vi "DetectorVI.vi"(8 "error in":errorcluster, 9 "Visible Temp Controls":bool=TRUE, 10 "ControlQueue":refnum<queue>, 11 "Detector.lvclass":refnum<class "Detector.lvclass">) -> (0 "error out":errorcluster)   [LabVIEW 2015, in "Detector.lvclass"]
uses:
  Detector.lvclass
  controls/SliderSD.ctl
  dependecies/ControlsVIs/Clusters-def/Message types.ctl
  Controls-refs_CLIENT.ctl
  Detector.lvclass/Detector.ctl
  GeneralFunctionality/GeneralFunctionality.lvclass/GeneralFunctionality.ctl
  Message/Message.lvclass/Message.ctl
  dependecies/ControlsVIs/Clusters-def/Standard Command.ctl
  dependecies/ControlsVIs/Clusters-def/DAQmx-ELYSE_pulse_counter.ctl
  dependecies/ControlsVIs/Clusters-def/OSc-WCM_max_value.ctl
  dependecies/ControlsVIs/Clusters-def/OSc-Diodes.ctl
  dependecies/ControlsVIs/Clusters-def/Det-Read.ctl
  dependecies/ControlsVIs/Clusters-def/Parameters_measurement_def.ctl
  Write SC sum values ref.vi
  dependecies/globalVarII.vi
  Message/Message.lvclass
  Control/Control-Client/Control-Client.lvclass
  GeneralFunctionality/GeneralFunctionality.lvclass
  DAQmxTasks/DAQmxTaskContainer_General/DAQmxTaksContainer_General.lvclass
  Oscilloscope/Oscilloscope.lvclass
panel:
  in  "Tab Control":enum32{"Detector", "PhotoDiodes"}(tab)
  in  "waves slider":T1={434.19354838709677, 734.8387096774194} scale=240.824..813.9446 scale format="%#.1f"
  in  "# error":i32=10
  out "Error Meter":dbl(knob) scale=0.0..10.0
  out "#PP":i32
  out "Spectra":cluster{"wavelengths":dbl[], "Tableau":dbl[]}[](graph)
  out "OD":cluster{"wavelengths":dbl[], "Tableau":dbl[]}(graph)
  in  "BG-level":i32
  in  "SC sum values":i32[](array[numeric])
  in  "Zeros for VIS-NIR":i32
  in  "Save spectra":bool
  out "Termometer":i32(slide) caption="T, °C" scale=-50.0..50.0
  in  "Set T":i32=-35
  in  "ON/OFF Cool":bool
  out "delta O.D.":dbl
  out "Ref I0":dbl(slide) scale=0.0..10.0
  out "Signal I0":dbl(slide) scale=0.0..10.0
  out "Ref Ie":dbl(slide) scale=0.0..10.0
  out "Signal Ie":dbl(slide) scale=0.0..10.0
  in  "All":bool
  out "class name":string
  out "WCM max":dbl
  out "ELYSE pulses":dbl
  in  "# scans":i32=5 min=1 max=50 step=1
  in  "Read detector":bool
  out "Received command":string
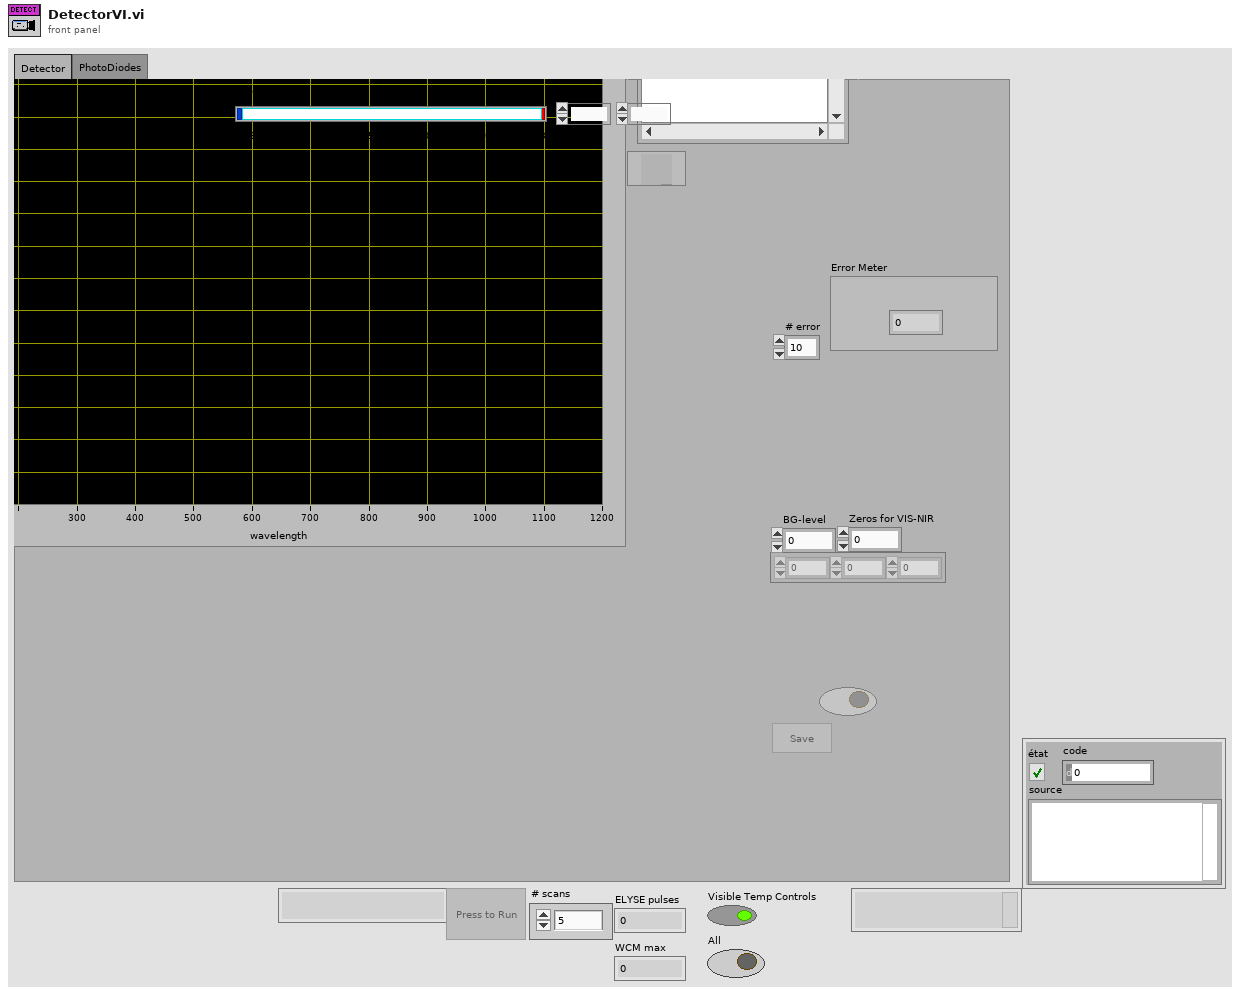
[diagram p1: front panel]
types:
  T1 = typedef "SliderSD.ctl" = cluster{dbl, dbl}
  T2 = typedef "Message types.ctl" = string
  T3 = typedef "Control-Client.lvclass/Controls-refs_CLIENT.ctl" = cluster{"ON/OFF Cool":refnum<vi>, "Save spectra":refnum<vi>, "Read detector":refnum<vi>, "# scans":refnum<vi>, "BG-level":refnum<vi>, "Set T":refnum<vi>, "Termometer":refnum<vi>, "Spectra":refnum<vi>, "Error Meter_ref":refnum<vi>, "waves slider":refnum<vi>}
  T4 = typedef "Standard Command.ctl" = cluster{"command":string, "data":variant}
  T5 = typedef "DAQmxTaksContainer_General.lvclass/DAQmx-ELYSE_pulse_counter.ctl" = cluster{"# counts":dbl}
  T6 = typedef "Oscilloscope.lvclass/OSc-WCM_max_value.ctl" = cluster{"WCM_max_value":dbl}
  T7 = typedef "Oscilloscope.lvclass/OSc-Diodes.ctl" = cluster{"I0":dbl, "Ie":dbl, "II0":dbl, "IIe":dbl, "BGI0":dbl, "BGIe":dbl, "BGII0":dbl, "BGIIe":dbl}
  T8 = typedef "Detector.lvclass/Det-Read.ctl" = cluster{"# scans":i32, "All":bool, "Parameters of measurement":T9}
  T9 = typedef "Parameters_measurement_def.ctl" = cluster{"ODmin":dbl, "ODmax":dbl, "Aq contol":enum32{"fixed", "automatic", "fixed-auto"}, "Wavelength_fix_index":i32, "WCM_limits":cluster{"WCM_min":dbl, "WCM_max":dbl, "WCM_value":dbl}, "WCM_corrections":bool, "#cycles max":i32}
  T10 = cluster{"closest index":i32, "closest index":i32}
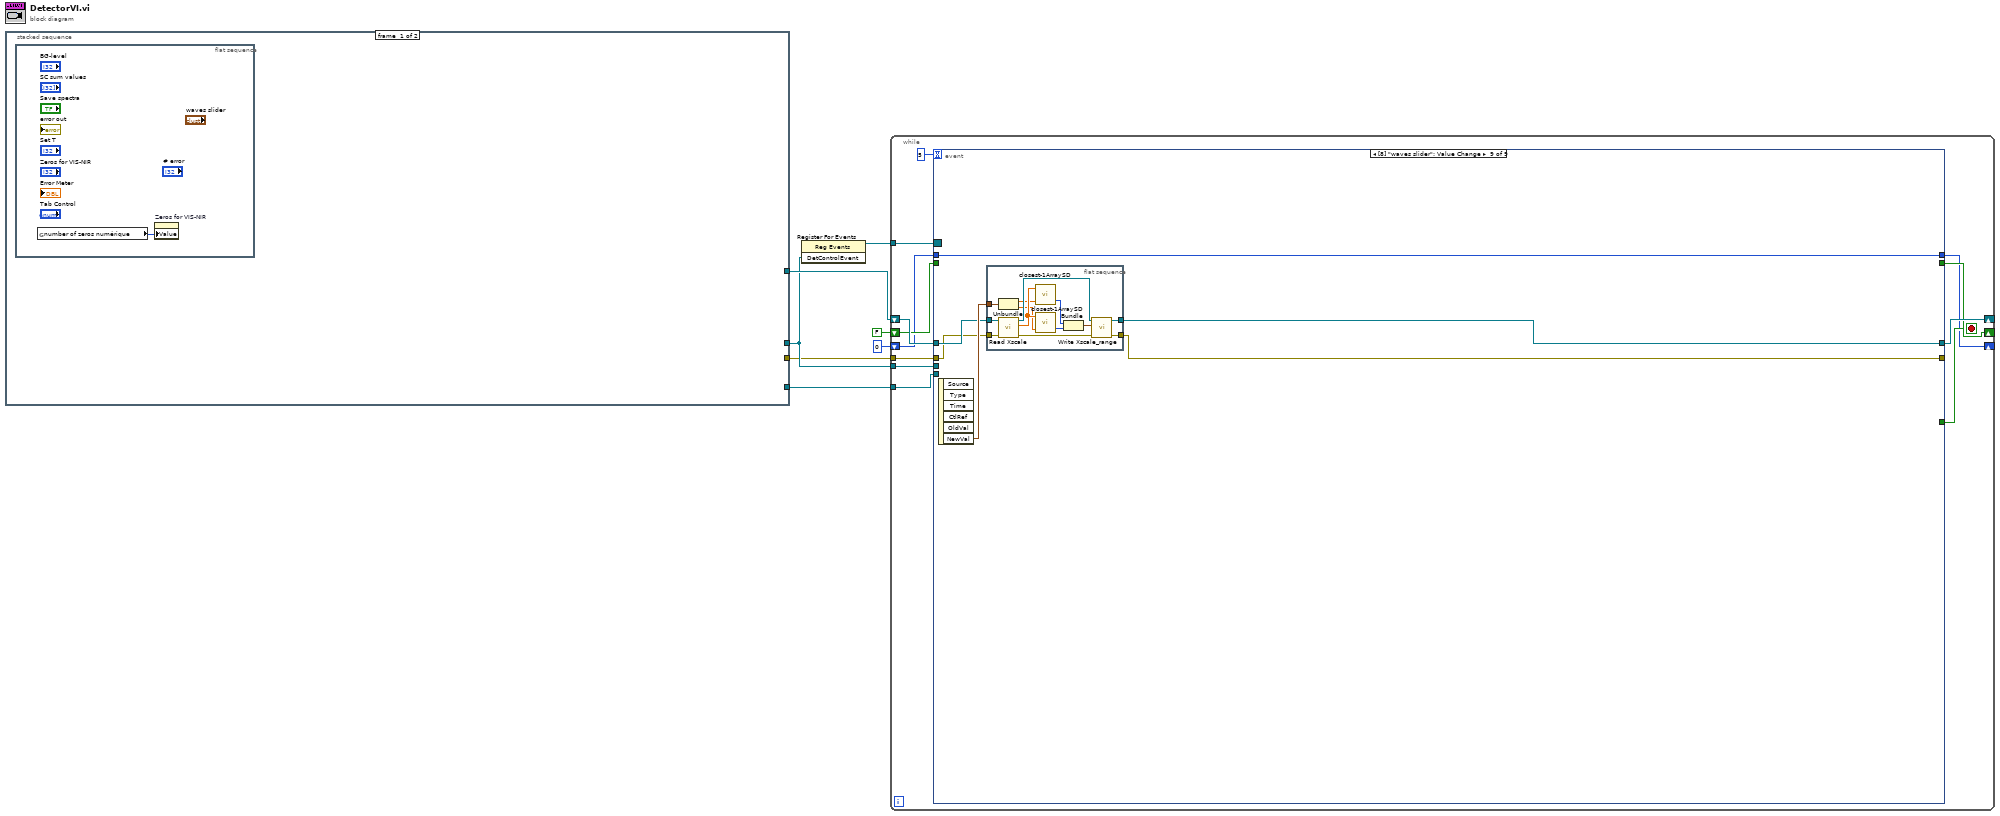
[diagram p0: block diagram]
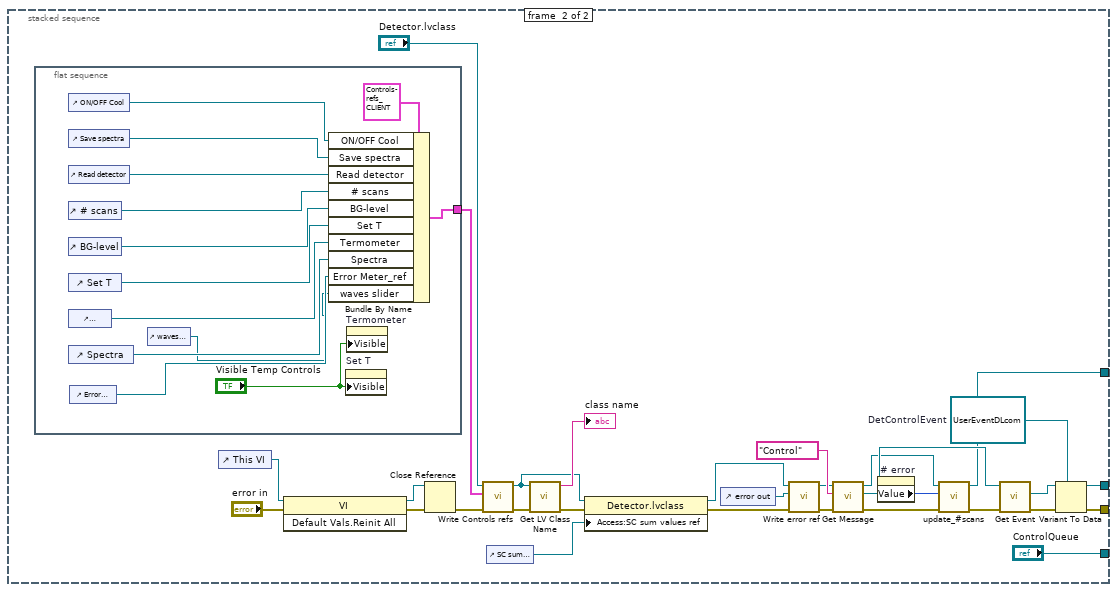
[diagram p2: hidden frame]
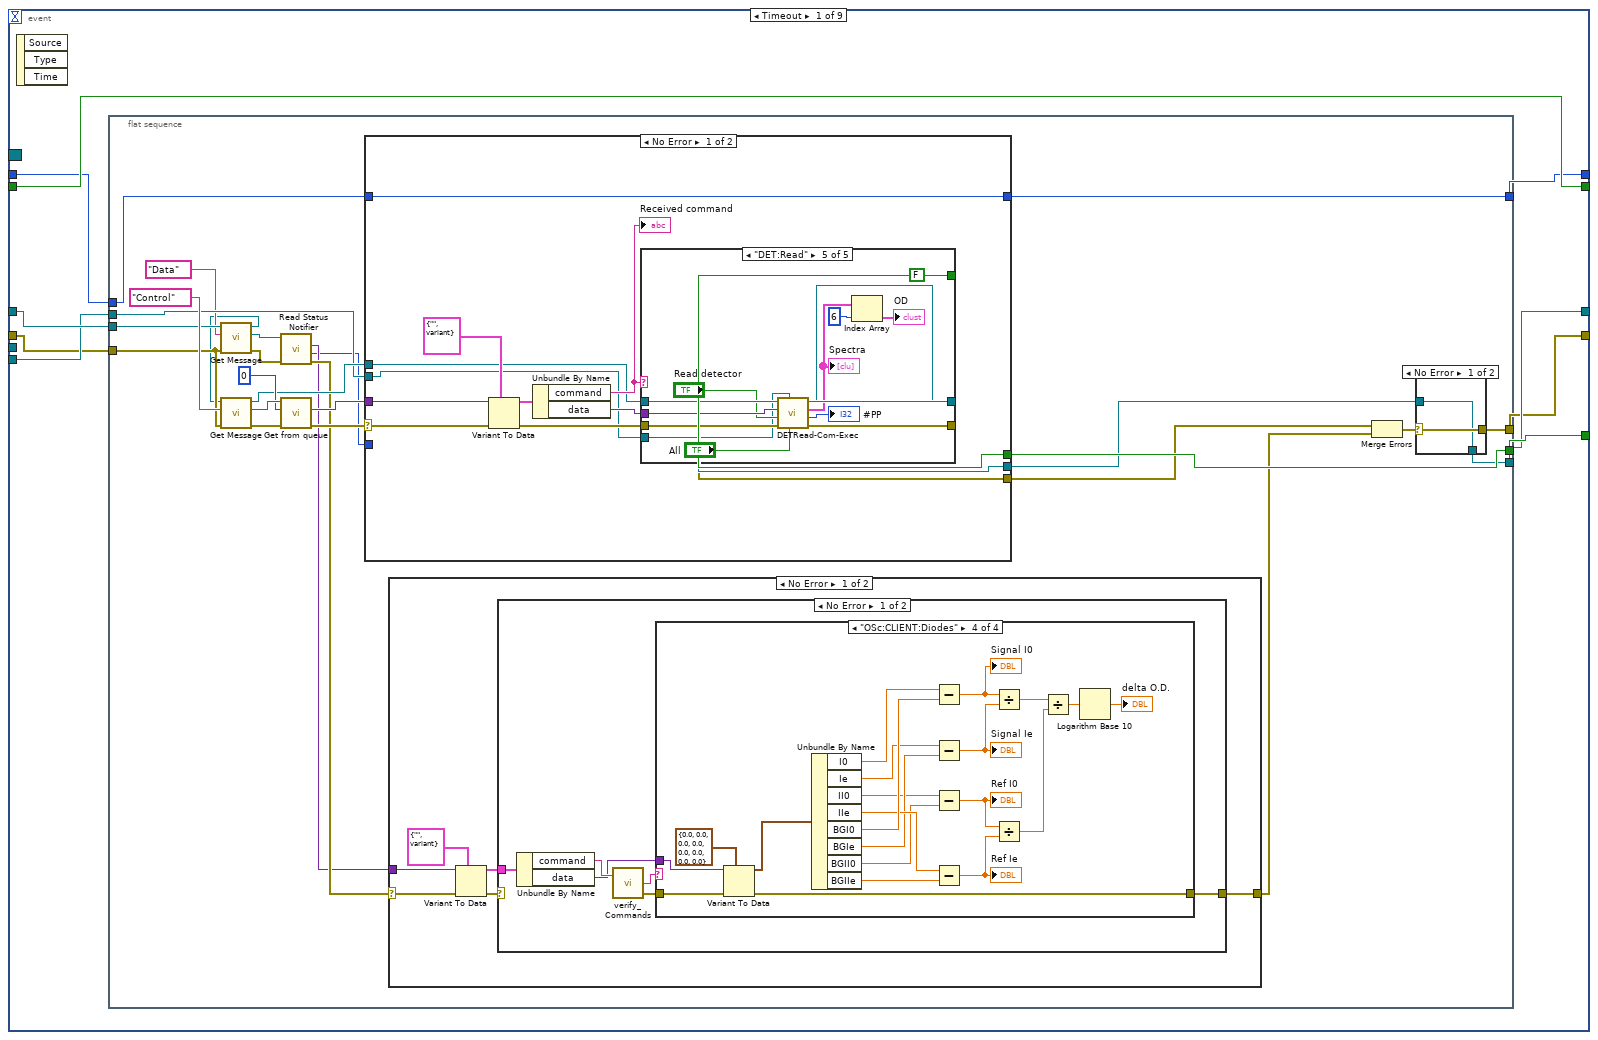
[diagram p3: hidden frame]
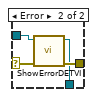
[diagram p4: hidden frame]
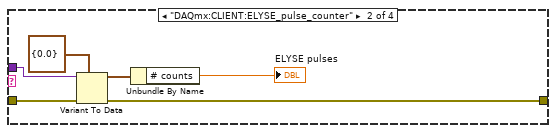
[diagram p6: hidden frame]
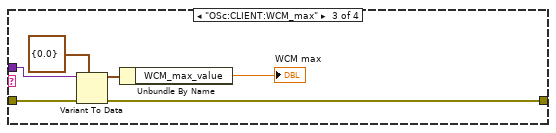
[diagram p7: hidden frame]
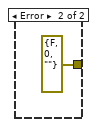
[diagram p8: hidden frame]
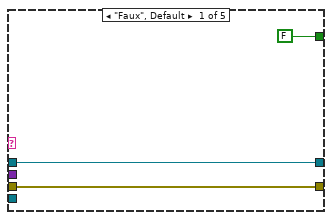
[diagram p10: hidden frame]
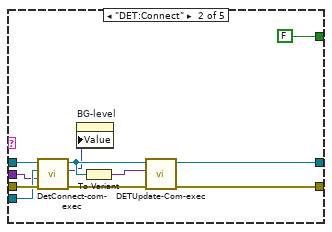
[diagram p11: hidden frame]
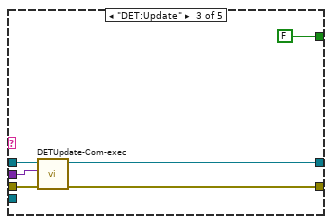
[diagram p12: hidden frame]
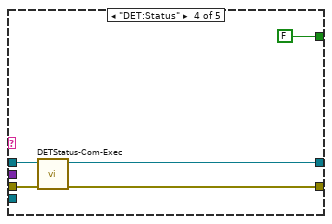
[diagram p13: hidden frame]
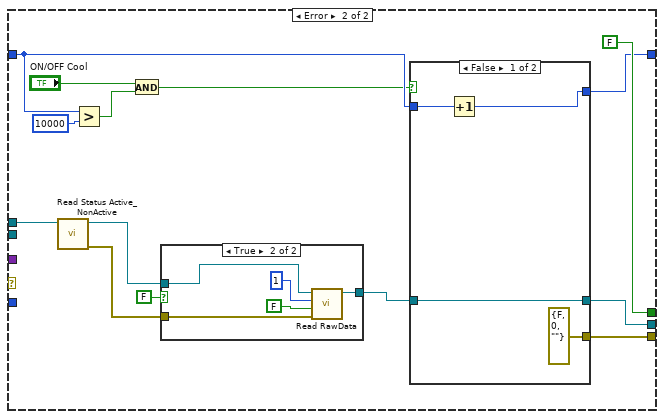
[diagram p14: hidden frame]
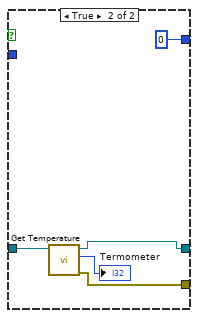
[diagram p16: hidden frame]
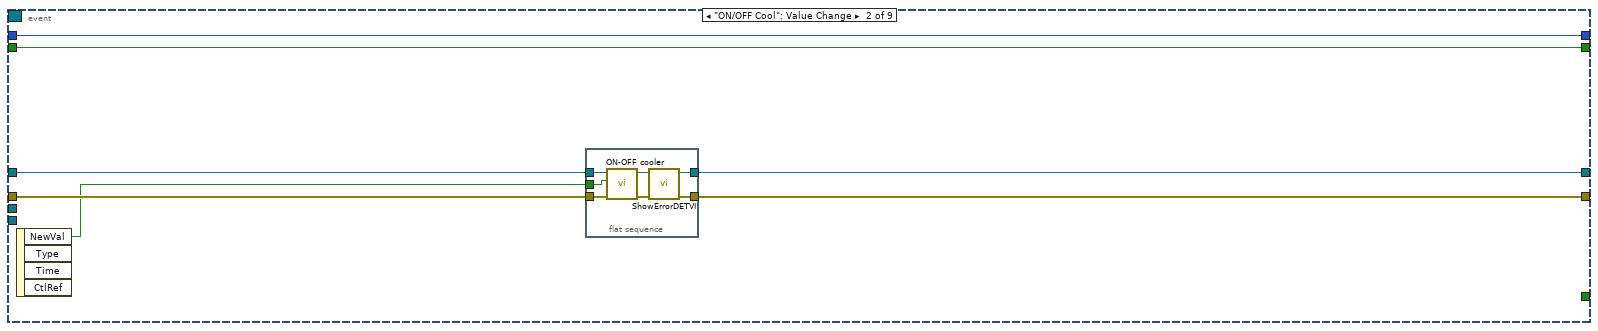
[diagram p17: hidden frame]
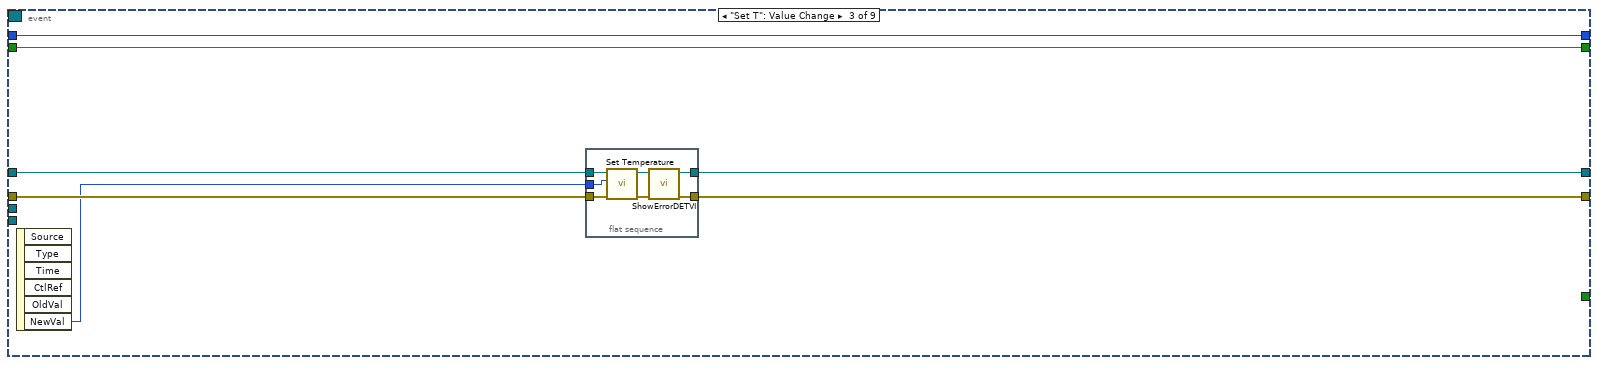
[diagram p18: hidden frame]
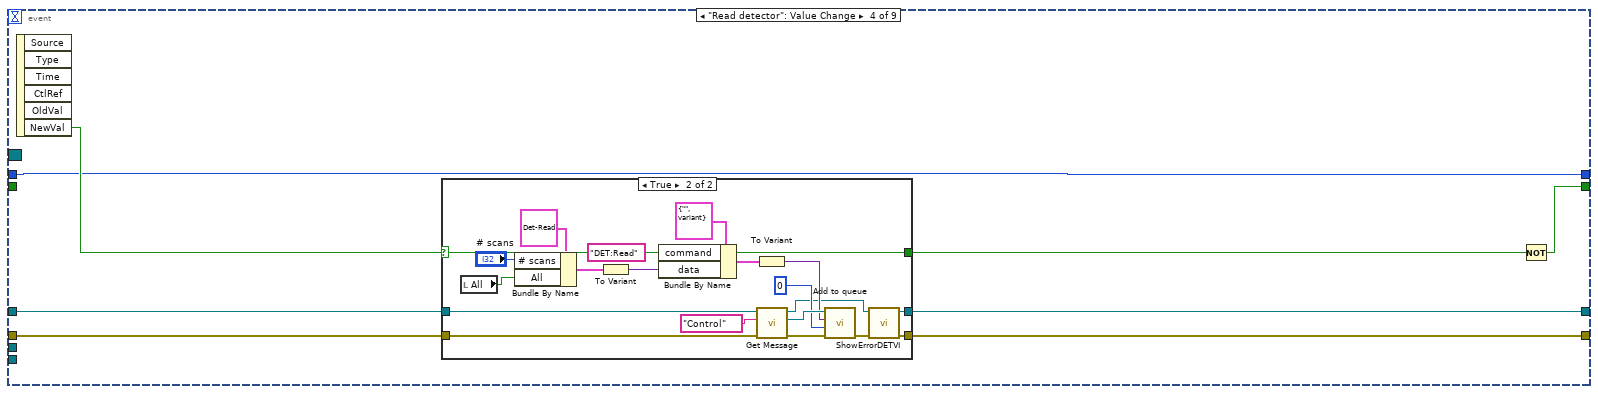
[diagram p19: hidden frame]
diagram:
  n1 = stacked-sequence {
    tunnel: [_ "ControlQueue"] -> w2
    tunnel: [_ w11] -> w7
    tunnel: [_ w29] -> w4
    tunnel: [_ w22] -> w3
    frame #0 {
      n2 = flat-sequence {
        frame #0 {
          n3 = global read "globalVarII.vi" "number of zeros numérique"() -> (w8:i32)
          n4 = property on="Zeros for VIS-NIR" class="DigNum (strict)"("Value"=w8) -> ()  [unwired: 2 in, 2 out]
        }
      }
    }
    frame #1 {
      w31 = refnum<user-event> refnum  # DetControlEvent
      n5 = flat-sequence {
        tunnel: [w43] -> w23
        frame #0 {
          n6 = control-ref of="ON/OFF Cool"() -> (w44:refnum<vi>)
          n7 = control-ref of="Save spectra"() -> (w45:refnum<vi>)
          n8 = control-ref of="Read detector"() -> (w46:refnum<vi>)
          n9 = control-ref of="# scans"() -> (w47:refnum<vi>)
          n10 = control-ref of="BG-level"() -> (w48:refnum<vi>)
          n11 = control-ref of="Set T"() -> (w49:refnum<vi>)
          n12 = control-ref of="Termometer"() -> (w50:refnum<vi>)
          n13 = control-ref of="Spectra"() -> (w42:refnum<vi>)
          n14 = control-ref of="Error Meter"() -> (w40:refnum<vi>)
          n15 = control-ref of="waves slider"() -> (w39:refnum<vi>)
          n16 = Bundle By Name(cluster=T3 {"ON/OFF Cool"=refnum, "Save spectra"=refnum, "Read detector"=refnum, "# scans"=refnum, "BG-level"=refnum, "Set T"=refnum, "Termometer"=refnum, "Spectra"=refnum, "Error Meter_ref"=refnum, "waves slider"=refnum} ("output cluster"), "ON/OFF Cool"=w44, "Save spectra"=w45, "Read detector"=w46, "# scans"=w47, "BG-level"=w48, "Set T"=w49, "Termometer"=w50, "Spectra"=w42, "Error Meter_ref"=w40, "waves slider"=w39) -> (w43:T3)
          n17 = property on="Set T" class="DigNum (strict)"("Visible"="Visible Temp Controls") -> ()  [unwired: 2 in, 2 out]
          n18 = property on="Termometer" class="Slide (strict)"("Visible"="Visible Temp Controls") -> ()  [unwired: 2 in, 2 out]
        }
      }
      n19 = control-ref of="This VI"() -> (w36:refnum<vi>)
      n20 = invoke class="VI" method="Default Vals.Reinit All"(reference=w36, error in="error in") -> (reference out=w37:refnum<vi>, error out=w38:errorcluster)  [unwired: 1 in, 1 out]
      n21 = Close Reference(reference=w37, error in (no error)=w38) -> (error out=w25:errorcluster)
      n22 = call "Write Controls refs.vi"("error in (no error)"=w25, "Controls refs"=w23, "Detector in"="Detector.lvclass") -> ("error out"=w19:errorcluster, "Detector out"=w18:refnum<class "Detector.lvclass">)  [unwired: 7 in]
      n23 = control-ref of="SC sum values"() -> (w14:refnum<vi>)
      n24 = call <vilib>:"Get LV Class Name.vi"("error in (no error)"=w19, "object"=w18) -> ("error out"=w15:errorcluster, "class name"=→"class name":string)  [unwired: 8 in]
      n25 = property class="Detector.lvclass"(reference=w18, error in=w15, "Access:SC sum values ref"=w14) -> (reference out=w17:refnum<class "Detector.lvclass">, error out=w16:errorcluster)
      n26 = control-ref of="error out"() -> (w26:refnum<vi>)
      n27 = call "Write error ref.vi"("error in (no error)"=w16, "error"=w26, "GeneralFunctionality in"=w17) -> ("error out"=w27:errorcluster, "GeneralFunctionality out"=w28:refnum<class "Detector.lvclass">)  [unwired: 7 in]
      n28 = call "Get Message.vi"("error in (no error)"=w27, "Message type"=T2 "Control", "GeneralFunctionality en entrée"=w28) -> ("error out"=w13:errorcluster, "Message.lvclass"=w32:refnum<class "Message.lvclass">, "GeneralFunctionality en sortie"=w10:refnum<class "Detector.lvclass">)  [unwired: 6 in]
      n29 = property on="# error" class="DigNum (strict)"() -> ("Value"=w9:i32)  [unwired: 2 in, 2 out]
      n30 = call "update_#scans.vi"("error in (no error)"=w13, "# scans"=w9, "Detector in"=w10) -> ("error out"=w12:errorcluster, "Detector out"=w11:refnum<class "Detector.lvclass">)  [unwired: 7 in]
      n31 = call "Get Event.vi"("error in (no error)"=w12, "Message en entrée"=w32) -> ("error out"=w20:errorcluster, "UserEventCommand"=w30:refnum<user-event>)  [unwired: 7 in, 1 out]
      n32 = Variant To Data(error in=w20, type=w31, Variant=w30) -> (data=w29:refnum<user-event>, error out=w22:errorcluster)
    }
  }
  n33 = register-events(w4) -> (reference out=w6:refnum<event-registration>)  [unwired: 2 in, 1 out]
  n34 = while {
    tunnel: w6 -> [w63]
    shift-right: [w60] -> _
    shift-left: w7 -> [w62]
    tunnel: w3 -> [w61]
    shift-right: [w59] -> _
    shift-left: FALSE ("Cooler status") -> [w58]
    tunnel: w4 -> [w57]
    tunnel: w2 -> [w56]
    shift-right: [w53] -> _
    shift-left: 0 -> [w54]
    stop <- w55 stop-if-true
    n35 = event shown="[8] \"waves slider\": Value Change" {
      selector: w63 -> [_ _ _ _ _ _ _ _ _]
      dyn-events: _ -> [_ _ _ _ _ _ _ _ _]
      timeout: 5 -> [_ _ _ _ _ _ _ _ _]
      tunnel: w62 -> [w71 w239 w253 w268 w300 w308 w315 w319 w365]
      tunnel: w61 -> [w67 w238 w252 w267 w299 w307 w314 w317 w364]
      tunnel: [w66 w234 w248 w266 w294 w307 w313 w316 w367] -> _
      tunnel: [w68 w235 w249 w262 w293 w308 w312 w319 w368] -> w60
      tunnel: [w72 w236 w250 w263 w297 _ _ _ _] -> w59
      tunnel: w58 -> [w72 w236 w250 _ w297 _ _ _ _]
      tunnel: w57 -> [_ _ _ _ w296 _ _ _ _]
      tunnel: w56 -> [w70 _ _ _ w295 _ _ _ _]
      tunnel: [w69 _ _ _ _ _ _ _ _] -> w55
      tunnel: w54 -> [w65 w233 w247 w261 w292 w306 w310 w320 w363]
      tunnel: [w64 w233 w247 w261 w292 w306 w310 w320 w363] -> w53
      event Timeout {
        n36 = event-data() -> ()  [unwired: 1 in, 3 out]
        n37 = flat-sequence {
          tunnel: w71 -> [w87]
          tunnel: w70 -> [w91]
          tunnel: [w90] -> w69
          tunnel: [w75] -> w68
          tunnel: [w78] -> w66
          tunnel: w67 -> [w86]
          tunnel: w65 -> [w89]
          tunnel: [w88] -> w64
          frame #0 {
            n38 = call "Get Message.vi"("error in (no error)"=w86, "Message type"=T2 "Data", "GeneralFunctionality en entrée"=w87) -> ("error out"=w84:errorcluster, "Message.lvclass"=w81:refnum<class "Message.lvclass">, "GeneralFunctionality en sortie"=w73:refnum<class "Detector.lvclass">)  [unwired: 6 in]
            n39 = call "Get Message.vi"("error in (no error)"=w86, "Message type"=T2 "Control", "GeneralFunctionality en entrée"=w73) -> ("error out"=w97:errorcluster, "Message.lvclass"=w96:refnum<class "Message.lvclass">, "GeneralFunctionality en sortie"=w92:refnum<class "Detector.lvclass">)  [unwired: 6 in]
            n40 = call "Read Status Notifier.vi"("error in (no error)"=w84, "Message in"=w81) -> ("error out"=w83:errorcluster, "nb en attente"=w74:i32, "latest notification"=w82:variant)  [unwired: 6 in, 1 out]
            n41 = call "Get from queue.vi"("error in (no error)"=w97, "timeout in ms (-1)"=0, "Message in"=w96) -> ("error out"=w93:errorcluster, "Data"=w94:variant)  [unwired: 5 in, 2 out]
            n42 = case shown="No Error" w93 {
              selector: w93 -> [w165 _]
              tunnel: w94 -> [w160 _]
              tunnel: [w153 w210] -> w80
              tunnel: [w159 FALSE] -> w90
              tunnel: [w154 w209] -> w76
              tunnel: w92 -> [w157 w207]
              tunnel: w91 -> [w156 _]
              tunnel: w89 -> [w155 w215]
              tunnel: [w155 w214] -> w88
              tunnel: w74 -> [_ _]
              frame No Error {
                n43 = Variant To Data(error in=w165, type=T4 {"command"="", "data"=variant} ("input cluster"), Variant=w160) -> (data=w163:T4, error out=w161:errorcluster)
                n44 = Unbundle By Name(w163) -> ("command"=w158:string, "data"=w162:variant)
                "Received command" <- w158
                n45 = case shown="\"DET:Read\"" w158 {
                  tunnel: [w168 w173 w181 w187 w202] -> w153
                  tunnel: [FALSE FALSE FALSE FALSE FALSE] -> w159
                  tunnel: w162 -> [_ w175 w183 _ w198]
                  tunnel: w161 -> [w168 w178 w182 w186 w203]
                  tunnel: [w166 w172 w180 w188 w201] -> w154
                  tunnel: w157 -> [w166 w177 w184 w189 w200]
                  tunnel: w156 -> [_ w176 _ _ w196]
                  frame "Faux", Default {
                  }
                  frame "DET:Connect" {
                    n46 = call "DetConnect-com-exec.vi"("error in (no error)"=w178, "data"=w175, "ControlQueue"=w176, "Detector in"=w177) -> ("error out"=w174:errorcluster, "BG_level"=w169:i32, "Detector out"=w171:refnum<class "Detector.lvclass">)  [unwired: 5 in]
                    n47 = property on="BG-level" class="DigNum (strict)"("Value"=w169) -> ()  [unwired: 2 in, 2 out]
                    n48 = To Variant(anything=w171) -> (Variant=w170:variant)
                    n49 = call "DETUpdate-Com-exec.vi"("error in (no error)"=w174, "data"=w170, "Detector in"=w171) -> ("error out"=w173:errorcluster, "Detector out"=w172:refnum<class "Detector.lvclass">)  [unwired: 6 in, 1 out]
                  }
                  frame "DET:Update" {
                    n50 = call "DETUpdate-Com-exec.vi"("error in (no error)"=w182, "data"=w183, "Detector in"=w184) -> ("error out"=w181:errorcluster, "Detector out"=w180:refnum<class "Detector.lvclass">)  [unwired: 6 in, 1 out]
                  }
                  frame "DET:Status" {
                    n51 = call "DETStatus-Com-Exec.vi"("error in (no error)"=w186, "Detector in"=w189) -> ("error out"=w187:errorcluster, "Detector out"=w188:refnum<class "Detector.lvclass">)  [unwired: 8 in]
                  }
                  frame "DET:Read" {
                    n52 = call "DETRead-Com-Exec.vi"("All"="All", "Control queue"=w196, "entrée d'erreur (pas d'erreur)"=w203, "Forever"="Read detector", "data"=w198, "Detector en entrée"=w200) -> ("sortie d'erreur"=w202:errorcluster, "#PP"=→"#PP":i32, "Spectra"=w195:cluster{"wavelengths":dbl[], "Tableau":dbl[]}[], "Detector out"=w201:refnum<class "Detector.lvclass">)  [unwired: 2 in]
                    "Spectra" <- w195
                    n53 = Index Array(array=w195, index=6 ("indice")) -> (element=→"OD":cluster{"wavelengths":dbl[], "Tableau":dbl[]})
                  }
                }
              }
              frame Error {
                n54 = call "Read Status Active_NonActive.vi"("GeneralFunctionality in"=w207) -> ("error out"=w205:errorcluster, "GeneralFunctionality out"=w206:refnum<class "Detector.lvclass">)  [unwired: 8 in, 1 out]
                n55 = Greater?(x=w215, y=10000) -> (0:w213:bool)
                n56 = And(x="ON/OFF Cool", y=w213) -> (x .and. y?=w211:bool)
                n57 = case shown="True" FALSE {
                  tunnel: [w218 w222] -> w208
                  tunnel: w206 -> [w218 w220]
                  tunnel: w205 -> [_ w219]
                  frame False {
                  }
                  frame True {
                    n58 = call-dynamic "Read RawData.vi"("error in (no error)"=w219, "WCM_max_value"=FALSE, "# of scans"=1, "Detector in"=w220) -> ("Detector out"=w222:refnum<class "Detector.lvclass">)  [unwired: 3 in, 4 out]
                  }
                }
                n59 = case shown="False" w211 {
                  tunnel: w215 -> [w227 _]
                  tunnel: [w226 0] -> w214
                  tunnel: w208 -> [w224 w230]
                  tunnel: [errorcluster {"status"=FALSE, "code"=0, "source"=""} ("error out") w228] -> w210
                  tunnel: [w224 w229] -> w209
                  frame False {
                    n60 = Increment(x=w227) -> (x+1=w226:i32)
                  }
                  frame True {
                    n61 = call-dynamic "Get Temperature.vi"("Detector in"=w230) -> ("error out"=w228:errorcluster, "Temperature"=→"Termometer":i32, "Detector out"=w229:refnum<class "Detector.lvclass">)  [unwired: 8 in]
                  }
                }
              }
            }
            n62 = case shown="No Error" w83 {
              selector: w83 -> [w107 w152]
              tunnel: w82 -> [w108 _]
              tunnel: [w106 w152] -> w77
              frame No Error {
                n63 = Variant To Data(error in=w107, type=T4 {"command"="", "data"=variant} ("input cluster"), Variant=w108) -> (data=w110:T4, error out=w105:errorcluster)
                n64 = case shown="No Error" w105 {
                  tunnel: w110 -> [w116 _]
                  tunnel: [w111 errorcluster {"status"=FALSE, "code"=0, "source"=""} ("error out")] -> w106
                  frame No Error {
                    n65 = Unbundle By Name(w116) -> ("command"=w115:string, "data"=w112:variant)
                    n66 = call "verify_Commands.vi"("Command"=w115) -> ("Command out"=w114:string, "error out"=w113:errorcluster)  [unwired: 1 in, 1 out]
                    n67 = case shown="\"OSc:CLIENT:Diodes\"" w114 {
                      tunnel: w113 -> [w117 w123 w129 w150]
                      tunnel: [w117 w118 w127 w148] -> w111
                      tunnel: w112 -> [_ w122 w128 w149]
                      frame "Error", Default {
                      }
                      frame "DAQmx:CLIENT:ELYSE_pulse_counter" {
                        n68 = Variant To Data(error in=w123, type=T5 {"# counts"=0.0} ("OSc:Read"), Variant=w122) -> (data=w120:T5, error out=w118:errorcluster)
                        n69 = Unbundle By Name(w120) -> ("# counts"=→"ELYSE pulses":dbl)
                      }
                      frame "OSc:CLIENT:WCM_max" {
                        n70 = Variant To Data(error in=w129, type=T6 {"WCM_max_value"=0.0} ("ELYSE pulses counter"), Variant=w128) -> (data=w125:T6, error out=w127:errorcluster)
                        n71 = Unbundle By Name(w125) -> ("WCM_max_value"=→"WCM max":dbl)
                      }
                      frame "OSc:CLIENT:Diodes" {
                        n72 = Variant To Data(error in=w150, type=T7 {"I0"=0.0, "Ie"=0.0, "II0"=0.0, "IIe"=0.0, "BGI0"=0.0, "BGIe"=0.0, "BGII0"=0.0, "BGIIe"=0.0} ("Diodes"), Variant=w149) -> (data=w147:T7, error out=w148:errorcluster)
                        n73 = Unbundle By Name(w147) -> ("I0"=w141:dbl, "Ie"=w133:dbl, "II0"=w131:dbl, "IIe"=w136:dbl, "BGI0"=w140:dbl, "BGIe"=w132:dbl, "BGII0"=w130:dbl, "BGIIe"=w135:dbl)
                        n74 = Subtract(x=w141, y=w140) -> (x-y=w139:dbl)
                        "Signal I0" <- w139
                        n75 = Subtract(x=w133, y=w132) -> (x-y=w138:dbl)
                        "Signal Ie" <- w138
                        n76 = Subtract(x=w131, y=w130) -> (x-y=w137:dbl)
                        "Ref I0" <- w137
                        n77 = Subtract(x=w136, y=w135) -> (x-y=w134:dbl)
                        "Ref Ie" <- w134
                        n78 = Divide(x=w139, y=w138) -> (x/y=w143:dbl)
                        n79 = Divide(x=w137, y=w134) -> (x/y=w142:dbl)
                        n80 = Divide(x=w143, y=w142) -> (x/y=w144:dbl)
                        n81 = Logarithm Base 10(1:w144) -> (0:→"delta O.D.":dbl)
                      }
                    }
                  }
                  frame Error {
                  }
                }
              }
              frame Error {
              }
            }
            n82 = Merge Errors(w80, w77) -> (w79:errorcluster)
            n83 = case shown="No Error" w79 {
              selector: w79 -> [w100 w104]
              tunnel: [w100 w103] -> w78
              tunnel: w76 -> [w99 w102]
              tunnel: [w99 w101] -> w75
              frame No Error {
              }
              frame Error {
                n84 = call "ShowErrorDETVI.vi"("error in (no error)"=w104, "Detector in"=w102) -> ("error out"=w103:errorcluster, "Detector out"=w101:refnum<class "Detector.lvclass">)  [unwired: 8 in]
              }
            }
          }
        }
      }
      event "ON/OFF Cool": Value Change {
        n85 = event-data() -> ("NewVal"=w237:bool)  [unwired: 1 in, 3 out]
        n86 = flat-sequence {
          tunnel: w239 -> [w246]
          tunnel: w238 -> [w245]
          tunnel: w237 -> [w244]
          tunnel: [w241] -> w235
          tunnel: [w240] -> w234
          frame #0 {
            n87 = call-dynamic "ON-OFF cooler.vi"("error in (no error)"=w245, "ON/OFF"=w244, "Detector in"=w246) -> ("error out"=w243:errorcluster, "Detector out"=w242:refnum<class "Detector.lvclass">)  [unwired: 7 in]
            n88 = call "ShowErrorDETVI.vi"("error in (no error)"=w243, "Detector in"=w242) -> ("error out"=w240:errorcluster, "Detector out"=w241:refnum<class "Detector.lvclass">)  [unwired: 8 in]
          }
        }
      }
      event "Set T": Value Change {
        n89 = event-data() -> ("NewVal"=w251:i32)  [unwired: 1 in, 5 out]
        n90 = flat-sequence {
          tunnel: w253 -> [w260]
          tunnel: w252 -> [w259]
          tunnel: w251 -> [w258]
          tunnel: [w255] -> w249
          tunnel: [w254] -> w248
          frame #0 {
            n91 = call-dynamic "Set Temperature.vi"("error in (no error)"=w259, "Numeric Control"=w258, "Detector in"=w260) -> ("error out"=w257:errorcluster, "Detector out"=w256:refnum<class "Detector.lvclass">)  [unwired: 7 in]
            n92 = call "ShowErrorDETVI.vi"("error in (no error)"=w257, "Detector in"=w256) -> ("error out"=w254:errorcluster, "Detector out"=w255:refnum<class "Detector.lvclass">)  [unwired: 8 in]
          }
        }
      }
      event "Read detector": Value Change {
        n93 = event-data() -> ("NewVal"=w265:bool)  [unwired: 1 in, 5 out]
        n94 = case shown="True" w265 {
          selector: w265 -> [w270 w291]
          tunnel: w268 -> [w269 w288]
          tunnel: w267 -> [w271 w287]
          tunnel: [w271 w276] -> w266
          tunnel: [w270 w291] -> w264
          tunnel: [w269 w274] -> w262
          frame False {
          }
          frame True {
            n95 = local read "All"() -> (w272:bool)
            n96 = Bundle By Name(cluster=T8 {"# scans"=0, "All"=FALSE, "Parameters of measurement"={"ODmin"=0.0, "ODmax"=0.0, "Aq contol"=enum."fixed", "Wavelength_fix_index"=640, "WCM_limits"={"WCM_min"=0.0, "WCM_max"=0.0, "WCM_value"=0.0}, "WCM_corrections"=FALSE, "#cycles max"=5}}, "# scans"="# scans", "All"=w272) -> (w282:T8)
            n97 = To Variant(anything=w282) -> (Variant=w281:variant)
            n98 = Bundle By Name(cluster=T4 {"command"="", "data"=variant} ("command"), "command"="DET:Read", "data"=w281) -> (w280:T4)
            n99 = To Variant(anything=w280) -> (Variant=w279:variant)
            n100 = call "Get Message.vi"("error in (no error)"=w287, "Message type"=T2 "Control", "GeneralFunctionality en entrée"=w288) -> ("error out"=w286:errorcluster, "Message.lvclass"=w285:refnum<class "Message.lvclass">, "GeneralFunctionality en sortie"=w275:refnum<class "Detector.lvclass">)  [unwired: 6 in]
            n101 = call "Add to queue.vi"("error in (no error)"=w286, "timeout in ms (-1)"=0, "Data"=w279, "Message in"=w285) -> ("error out"=w277:errorcluster)  [unwired: 6 in, 1 out]
            n102 = call "ShowErrorDETVI.vi"("error in (no error)"=w277, "Detector in"=w275) -> ("error out"=w276:errorcluster, "Detector out"=w274:refnum<class "Detector.lvclass">)  [unwired: 8 in]
          }
        }
        n103 = Not(x=w264) -> (.not. x?=w263:bool)
      }
      event "BG-level": Value Change {
        n104 = event-data() -> ("NewVal"=w298:i32)  [unwired: 1 in, 5 out]
        n105 = flat-sequence {
          tunnel: w300 -> [w302]
          tunnel: w299 -> [w303]
          tunnel: w298 -> [w301]
          tunnel: w296 -> [_]
          tunnel: w295 -> [_]
          tunnel: [w305] -> w294
          tunnel: [w304] -> w293
          frame #0 {
            n106 = call-dynamic "Write BG_level.vi"("error in (no error)"=w303, "BG_level"=w301, "Detector in"=w302) -> ("error out"=w305:errorcluster, "Detector out"=w304:refnum<class "Detector.lvclass">)  [unwired: 7 in]
          }
        }
      }
      event "Zeros for VIS-NIR": Value Change {
        n107 = event-data() -> ("NewVal"=w309:i32)  [unwired: 1 in, 5 out]
        n108 = global write "globalVarII.vi" "number of zeros numérique"(w309) -> ()
      }
      event "# error": Value Change {
        n109 = event-data() -> ("NewVal"=w311:i32)  [unwired: 1 in, 5 out]
        n110 = call "update_#scans.vi"("error in (no error)"=w314, "# scans"=w311, "Detector in"=w315) -> ("error out"=w313:errorcluster, "Detector out"=w312:refnum<class "Detector.lvclass">)  [unwired: 7 in]
      }
      event "Spectra": Shortcut Menu Selection (User) {
        n111 = event-data() -> ("ItemTag"=w318:string)  [unwired: 1 in, 7 out]
        n112 = flat-sequence {
          tunnel: w318 -> [w335]
          tunnel: w317 -> [w322]
          tunnel: [w321] -> w316
          frame #0 {
            w325 = "%f" ("format string")
            n113 = property on="Spectra" class="XYGraph (strict)"() -> ("Value"=w323:cluster{"wavelengths":dbl[], "Tableau":dbl[]}[])  [unwired: 2 in, 2 out]
            n114 = case shown="\"Copy all\", Default" w335 {
              tunnel: [w339 w361] -> w331
              tunnel: w323 -> [w336 w357]
              tunnel: [w337 w359] -> w328
              frame "Copy all", Default {
                n115 = for {
                  shift-right: [w346] -> w339
                  shift-left: dbl[][] [] ("appended array") -> [w350]
                  tunnel: w336 -> [w349] mode=indexing
                  shift-right: [w344] -> w337
                  shift-left: string[] [] ("Plots names") -> [w345]
                  i -> [w341]
                  n116 = Unbundle(w349) -> ("wavelengths"=w348:dbl[], "Tableau"=w347:dbl[])
                  n117 = Number To Decimal String(number=w341) -> (decimal integer string=w342:string)  [unwired: 1 in]
                  n118 = Insert Into Array(array=w345, new element #1="X" ("element"), new element #2=w342) -> (w344:string[])  [unwired: 1 in]
                  n119 = Build Array (concatenate)(w350, w348, w347) -> (w346:dbl[][])
                }
              }
              frame "Copy last" {
                n120 = Array Size(array=w357) -> (size(s)=w358:i32)
                n121 = Decrement(x=w358) -> (x-1=w351:i32)
                n122 = Index Array(array=w357, index=w351) -> (element=w352:cluster{"wavelengths":dbl[], "Tableau":dbl[]})
                n123 = Unbundle(w352) -> ("wavelengths"=w356:dbl[], "Tableau"=w355:dbl[])
                n124 = Number To Decimal String(number=w351) -> (decimal integer string=w353:string)  [unwired: 1 in]
                n125 = Insert Into Array(array=string[] [] ("Plots names"), new element #1="X" ("element"), new element #2=w353) -> (w359:string[])  [unwired: 1 in]
                n126 = Build Array (concatenate)(dbl[][] [] ("appended array"), w356, w355) -> (w361:dbl[][])
              }
            }
            n127 = Transpose 2D Array(2D array=w331) -> (transposed array=w330:dbl[][])
            n128 = Array To Spreadsheet String(array=w328, 3:w325) -> (spreadsheet string=w327:string)  [unwired: 1 in]
            n129 = Array To Spreadsheet String(array=w330, 3:w325) -> (spreadsheet string=w326:string)  [unwired: 1 in]
            n130 = Concatenate Strings(w327, w326) -> (w324:string)
            n131 = call "replace_in_stringSD.vi"("error in (no error)"=w322, "replaced to.."=".", "characters to replace"="[,]+", "input string"=w324) -> ("error out"=w329:errorcluster, "output string"=w332:string)
            n132 = invoke class="App" method="Clipboard.Write"(error in=w329, "Param 0"=w332) -> (error out=w321:errorcluster)  [unwired: 2 in, 3 out]
          }
        }
      }
      event Value Change {
        n133 = event-data() -> ("NewVal"=w366:T1)  [unwired: 1 in, 5 out]
        n134 = flat-sequence {
          tunnel: [w381] -> w368
          tunnel: [w380] -> w367
          tunnel: w366 -> [w371]
          tunnel: w365 -> [w379]
          tunnel: w364 -> [w378]
          frame #0 {
            n135 = Unbundle(w371) -> (w370:dbl, w369:dbl)
            n136 = call "Read Xscale.vi"("error in (no error)"=w378, "Detector en entrée"=w379) -> ("error out"=w372:errorcluster, "Xscale"=w375:dbl[], "Detector en sortie"=w377:refnum<class "Detector.lvclass">)  [unwired: 7 in]
            n137 = call "closest-1ArraySD.vi"("desired element"=w370, "1D Array"=w375) -> ("closest index"=w376:i32)  [unwired: 1 in, 1 out]
            n138 = call "closest-1ArraySD.vi"("desired element"=w369, "1D Array"=w375) -> ("closest index"=w374:i32)  [unwired: 1 in, 1 out]
            n139 = Bundle("closest index"=w376, "closest index"=w374) -> (w373:T10)  [unwired: 1 in]
            n140 = call "Write Xscale_range.vi"("error in (no error)"=w372, "Xscale_range"=w373, "Detector in"=w377) -> ("error out"=w380:errorcluster, "Detector out"=w381:refnum<class "Detector.lvclass">)  [unwired: 7 in]
          }
        }
      }
    }
  }
